vi "Run Game.vi"   [LabVIEW 2020]
uses:
  FormulaG/FormulaG App/FormulaG App.lvclass
panel:
  # "Run this VI to play!"
types:
  T1 = enum32{"Invalid", "Standard", "Closed", "Hidden", "Minimized", "Maximized"}
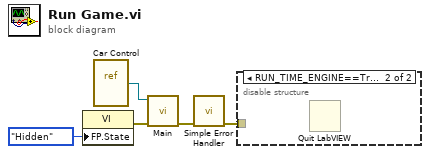
[diagram p0: block diagram]
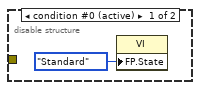
[diagram p2: hidden frame]
diagram:
  n1 = property class="VI"("FP.State"=T1."Hidden" ("Front Panel Window:State")) -> (error out=w3:errorcluster)  [unwired: 2 in, 1 out]
  n2 = vi-ref "Car Control.vi"() -> (w5:refnum<vi>)
  n3 = call "Main.vi"("error in (no error)"=w3, "Control VI"=w5) -> ("error out"=w2:errorcluster)  [unwired: 9 in]
  n4 = call <vilib>:"Simple Error Handler.vi"("error in (no error)"=w2) -> ("error out"=w1:errorcluster)  [unwired: 4 in, 4 out]
  n5 = disable-structure shown="RUN_TIME_ENGINE==True" {
    disable-tunnel: w1 -> [_ _]
    frame condition #0 (active) {
      n6 = property class="VI"("FP.State"=T1."Standard" ("Front Panel Window:State")) -> ()  [unwired: 2 in, 2 out]
    }
    frame condition #1 {
      n7 = Quit LabVIEW() -> ()  [unwired: 1 in]
    }
  }
